vi "blink led using shift register.vi"() -> ()   [LabVIEW 2018]
panel:
  in  "milliseconds to wait":u32=500
  in  "stop":bool
  out "Boolean":bool
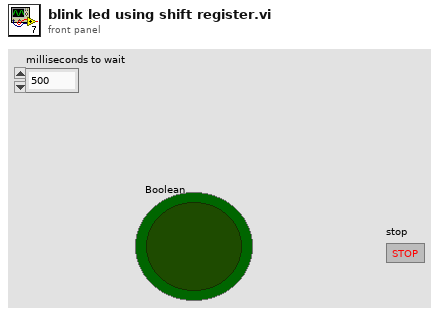
[diagram p1: front panel]
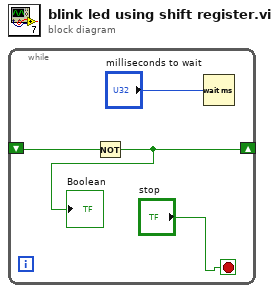
[diagram p0: block diagram]
diagram:
  n1 = while {
    shift-right: [w3] -> _
    shift-left: _ -> [w1]
    stop <- "stop" stop-if-true
    n2 = Not(x=w1) -> (.not. x?=w3:bool)
    "Boolean" <- w3
    n3 = Wait (ms)(milliseconds to wait="milliseconds to wait") -> ()  [unwired: 1 out]
  }
